vi "Create Test Results Stacked Bar Graph.vi"(6 "target image filepath":path, 8 "error in (no error)":errorcluster, 9 "labels":T2, 10 "test results":T1) -> (0 "error out":errorcluster, 2 "test results stacked bar graph":picture)   [LabVIEW 2019, in "Python Visualizations.lvlib"]
uses:
  Python Visualizations.lvlib
  pieplot_labels.ctl
  <vilib>/Utility/sysdir.llb/System Directory Type.ctl
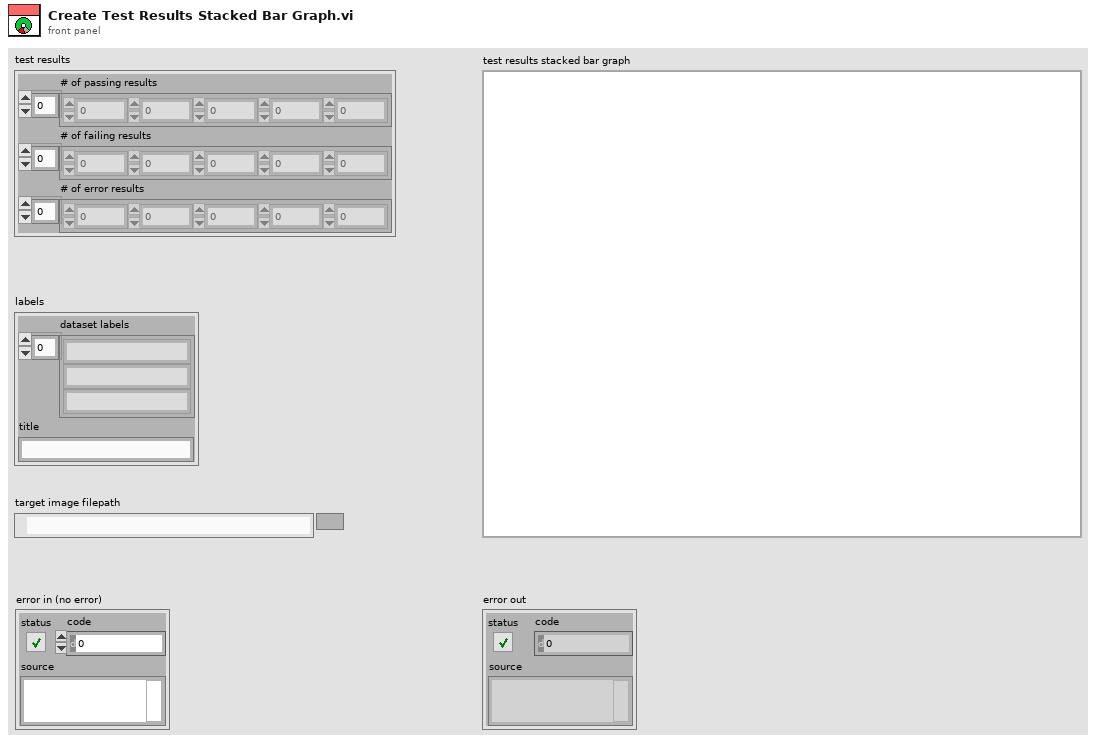
[diagram p1: front panel]
types:
  T1 = cluster{"# of passing results":dbl[], "# of failing results":dbl[], "# of error results":dbl[]}
  T2 = typedef "Python Visualizations.lvlib/pieplot_labels.ctl" = cluster{"dataset labels":string[], "title":string}
  T3 = typedef "System Directory Type.ctl" = i32
  T4 = typedef "imagedata.ctl" = cluster{"image type":i32, "image depth":i32, "image":u8[], "mask":u8[], "colors":u32[], "Rectangle":cluster{"left":i16, "top":i16, "right":i16, "bottom":i16}}
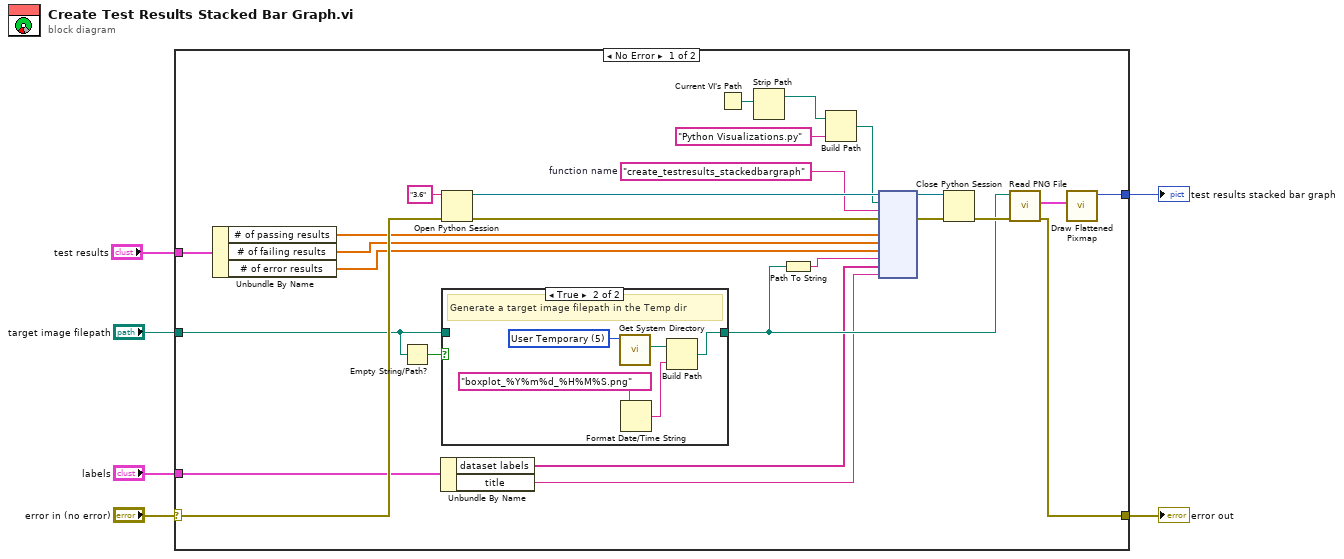
[diagram p0: block diagram]
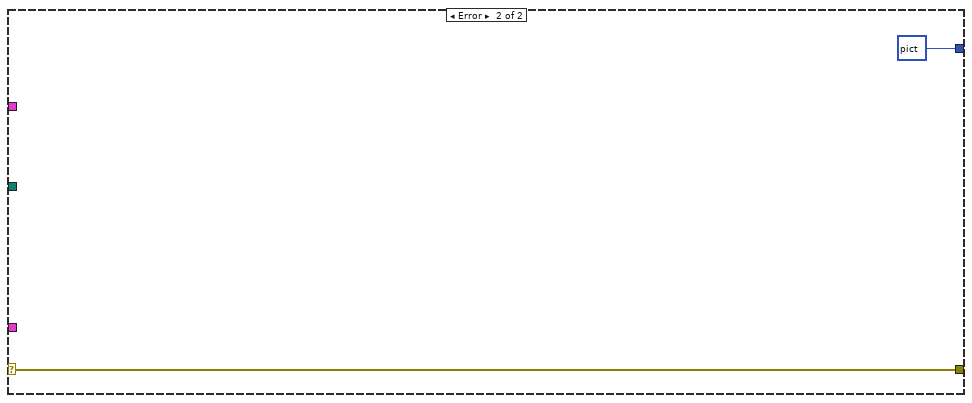
[diagram p3: hidden frame]
diagram:
  n1 = case shown="No Error" "error in (no error)" {
    selector: "error in (no error)" -> [w22 w40]
    tunnel: [w24 picture data[5B] ("new picture")] -> w6
    tunnel: [w21 w40] -> w4
    tunnel: "target image filepath" -> [w16 _]
    tunnel: "labels" -> [w14 _]
    tunnel: "test results" -> [w10 _]
    frame No Error {
      w28 = "create_testresults_stackedbargraph"  # function name
      n2 = Unbundle By Name(w10) -> ("# of passing results"=w9:dbl[], "# of failing results"=w8:dbl[], "# of error results"=w7:dbl[])
      n3 = Empty String/Path?(string/path=w16) -> (empty?=w17:bool)
      n4 = Unbundle By Name(w14) -> ("dataset labels"=w12:string[], "title"=w11:string)
      n5 = Open Python Session(python version="3.6" ("Python version"), 3:w22) -> (session out=w32:refnum<k35>, error out=w31:errorcluster)  [unwired: 1 in]
      n6 = case shown="True" w17 {
        tunnel: w16 -> [w33 _]
        tunnel: [w33 w34] -> w15
        frame False {
          # "Caller has specified a target image filepath"
        }
        frame True {
          w38 = T3 5 items=["User Home"=0, "User Desktop"=1, "User Documents"=2, "User Application Data"=3, "User Preferences"=4, "User Temporary"=5, "Public Documents"=6, "Public Application Data"=7, "Public Preferences"=8, "Public Cache"=13, "System Core Libraries"=9, "System Installed Libraries"=10, "Application Files"=11, "Boot Volume Root"=12] ("system directory type")
          # "Generate a target image filepath in the Temp dir"
          n7 = call <vilib>:"Get System Directory.vi"("system directory type"=w38) -> ("system directory"=w37:path)  [unwired: 10 in]
          n8 = Format Date/Time String(time format string (%c)="boxplot_%Y%m%d_%H%M%S.png") -> (date/time string=w35:string)  [unwired: 2 in]
          n9 = Build Path(base path=w37, name or relative path=w35) -> (appended path=w34:path)
        }
      }
      n10 = Current VI's Path() -> (path=w19:path)
      n11 = Strip Path(path=w19) -> (stripped path=w18:path)  [unwired: 1 out]
      n12 = Path To String(path=w15) -> (string=w13:string)
      n13 = Build Path(base path=w18, name or relative path="Python Visualizations.py") -> (appended path=w29:path)
      n14 = node(w32, w29, w28, w31, w9, w8, w7, w13, w12, w11) -> (w27:refnum<k35>, w26:errorcluster)  [unwired: 8 in, 2 out]
      n15 = Close Python Session(session in=w27, error in=w26) -> (11:w23:errorcluster)
      n16 = call <vilib>:"Read PNG File.vi"("error in (no error)"=w23, "path to PNG file"=w15) -> ("error out"=w21:errorcluster, "image data"=w25:T4)  [unwired: 7 in, 1 out]
      n17 = call <vilib>:"Draw Flattened Pixmap.vi"("image data"=w25) -> ("new picture"=w24:picture)  [unwired: 8 in]
    }
    frame Error {
    }
  }
  "error out" <- w4
  "test results stacked bar graph" <- w6
